vi "Climber Controller.vi"(8 "error in":errorcluster) -> ()   [LabVIEW 2019]
doc: "This VI executes continuously carrying out the current operation and responding to updates or new operations. It will often contain the timing or control code that is difficult to place directly in TeleOp. This VI generally opens all sensors and motors and isolates the rest of the robot code from knowing how the operations are carried out."
uses:
  <vilib>/Rock Robotics/WPI/Framework/Completion Status.ctl
  Climber Setpoints.ctl
  Climber Operations.ctl
  <vilib>/Rock Robotics/WPI/MotorControl/WPI_MotorControlDeviceRef.ctl
  <vilib>/Rock Robotics/WPI/MotorControl/WPI_MotorControlType.ctl
  <vilib>/Rock Robotics/SystemInterfaces/DIO/FPGA_DIOPWMChannel.ctl
  <vilib>/Rock Robotics/WPI/PWM/WPI_PWMDeadband.ctl
  <vilib>/Rock Robotics/SystemInterfaces/DIO/FPGA_DIOChannel.ctl
  <vilib>/Rock Robotics/WPI/ThirdParty/REV Robotics/SPARK MAX/Typedef/Spark MAX Limit Direction.ctl
panel:
  in  "Max Reverse Speed":dbl=-0.1
  out "Applied Output":dbl
  out "Sensor Velocity":dbl
  in  "Smart Position":dbl=40.0
  out "Sensor Position":dbl=-0.11904771625995636
  in  "Interactive Values":T1
  out "Current\nCmd":string="Started at  21:27:06.976\n: Extend Climb,  S 0.0, D 0.000000"
  in  "Buttons":cluster{"Execute Cmd":bool, "Abort Cmd":bool}
  out "Command Timing":cluster{"Start Time (ms)":u32, "Iterations":i32}={"Start Time (ms)"=7212987, "Iterations"=0}
  out "Status":T3
  # "Interactive Command: You may fill in the settings for a command\nand schedule it with the Execute button. You can observe and abort\nany command while fine tuning the code for the controller."
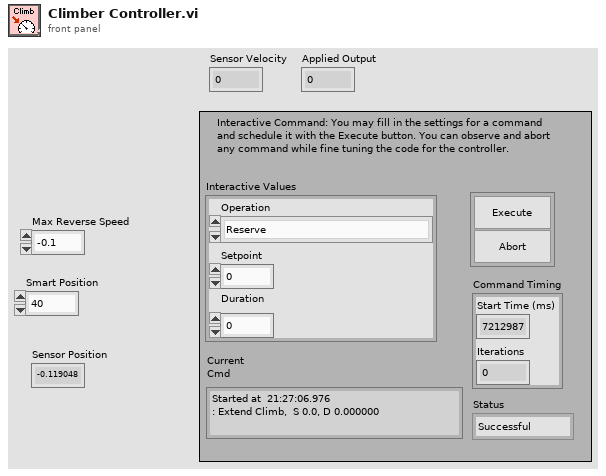
[diagram p1: front panel]
types:
  T1 = typedef "Climber Setpoints.ctl" = cluster{"Operation":T2, "Setpoint":dbl, "Duration":dbl}
  T2 = typedef "Climber Operations.ctl" = enum16{"Reserve", "Read Current", "Immediate", "Revert Climb", "Extend Climb"}
  T3 = typedef "Completion Status.ctl" = enum16{"Successful", "Aborted", "Incomplete"}
  T4 = typedef "Spark MAX Limit Direction.ctl" = enum16{"Forward Limit", "Reverse Limit"}
  T5 = typedef "WPI_MotorControlDeviceRef.ctl" = cluster{"DeviceStatus":errorcluster, "Type":T6, "PWM":cluster{"PWM Channel":T7, "DeadBand":T8}, "CAN":cluster{"Device Number":u8, "SetOutput VI Ref":variant, "GetOutput VI Ref":variant, "Enable VI Ref":variant, "Disable VI Ref":variant, "Data":variant}, "Invert":bool, "DIO PWM":cluster{"PWM \"Enable\" Channel":T7, "DIOChannel":T9, "PWM Rate":dbl}}
  T6 = typedef "WPI_MotorControlType.ctl" = enum16{"PWM", "CAN", "DIO PWM"}
  T7 = typedef "FPGA_DIOPWMChannel.ctl" = enum8{"PWM 0", "PWM 1", "PWM 2", "PWM 3", "PWM 4", "PWM 5", "PWM 6", "PWM 7", "PWM 8", "PWM 9", "PWM MXP 0", "PWM MXP 1", "PWM MXP 2", "PWM MXP 3", "PWM MXP 4", "PWM MXP 5", "PWM MXP 6", "PWM MXP 7", "PWM MXP 8", "PWM MXP 9", "Invalid"}
  T8 = typedef "WPI_PWMDeadband.ctl" = cluster{"Name":string, "maxPositivePwm":i32, "minPositivePwm":i32, "centerPwm":i32, "maxNegativePwm":i32, "minNegativePwm":i32, "angularRange":u16}
  T9 = typedef "FPGA_DIOChannel.ctl" = enum8{"DIO 0", "DIO 1", "DIO 2", "DIO 3", "DIO 4", "DIO 5", "DIO 6", "DIO 7", "DIO 8", "DIO 9", "DIO MXP 0", "DIO MXP 1", "DIO MXP 2", "DIO MXP 3", "DIO MXP 4", "DIO MXP 5", "DIO MXP 6", "DIO MXP 7", "DIO MXP 8", "DIO MXP 9", "DIO MXP 10", "DIO MXP 11", "DIO MXP 12", "DIO MXP 13", "DIO MXP 14", "DIO MXP 15", "SPI Port CS1", "SPI Port CS2", "SPI Port CS3", "SPI Port MISO", "SPI Port MOSI", "Invalid"}
  T10 = typedef "Command Status Info.ctl" = cluster{"Name":string, "Status":T3, "notifier out":T11}
  T11 = typedef "Completion Notifier.ctl" = refnum<notifier>
  T12 = cluster{"Current Command":T1, "Command Timing":cluster{"Start Time (ms)":u32, "Iterations":i32}, "Command Arguments":cluster{"Command Info":T10, "Description":string, "Default Command":T1, "queue out":refnum<queue>, "Subsystem Name":string}}
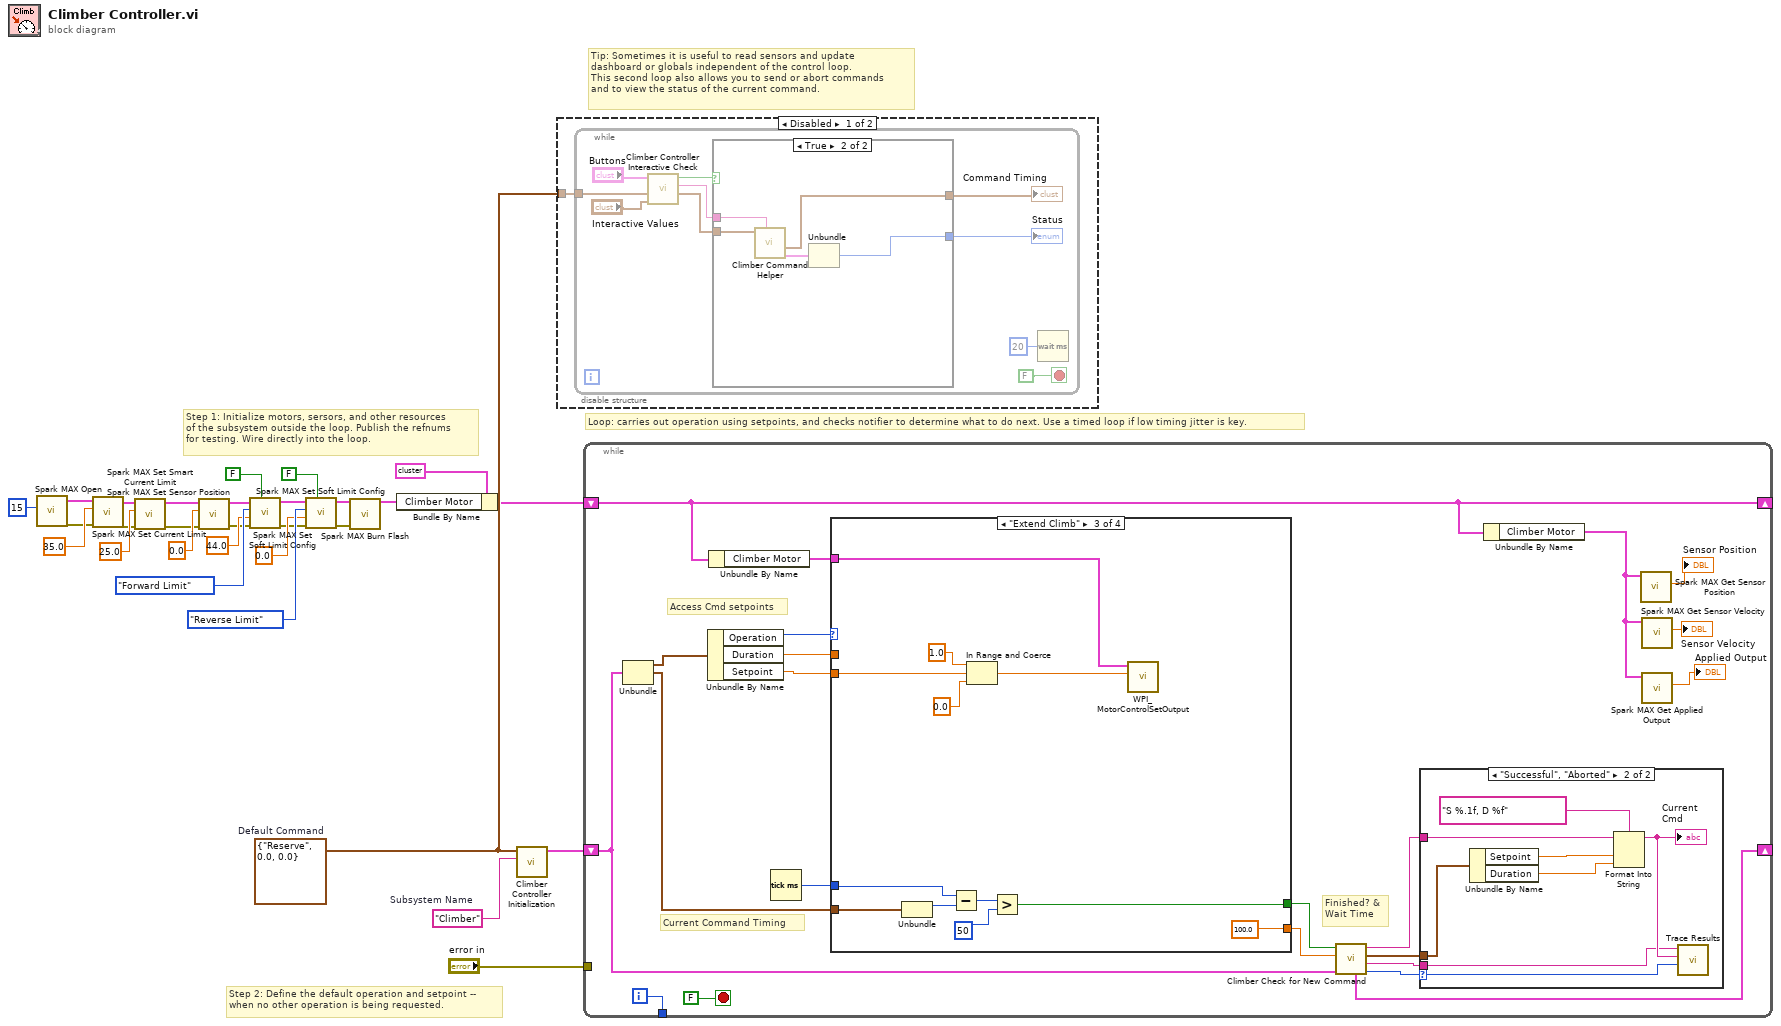
[diagram p0: block diagram]
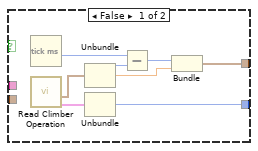
[diagram p2: hidden frame]
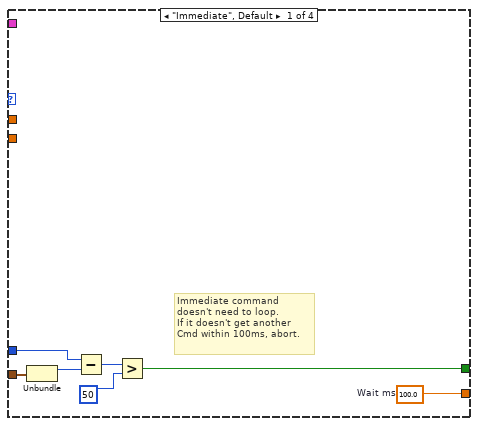
[diagram p5: hidden frame]
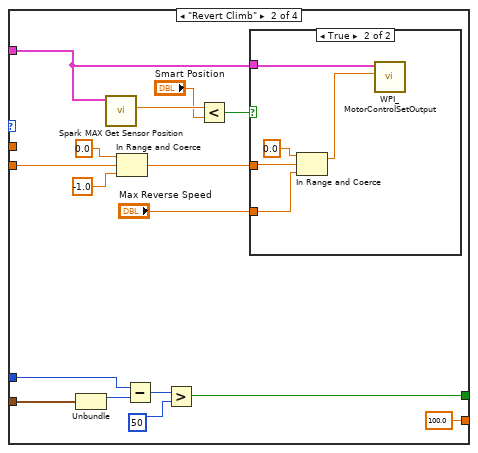
[diagram p6: hidden frame]
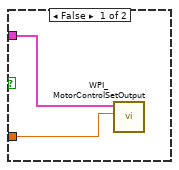
[diagram p7: hidden frame]
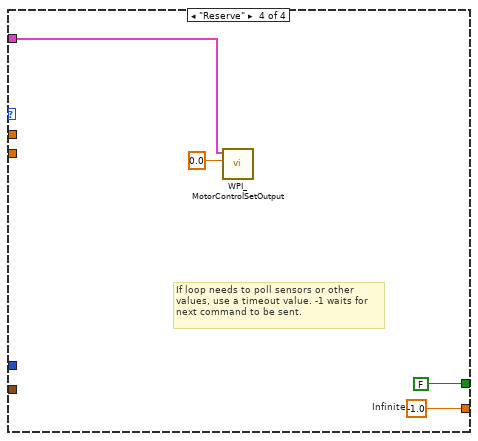
[diagram p8: hidden frame]
diagram:
  w26 = T1 {"Operation"=enum."Reserve", "Setpoint"=0.0, "Duration"=0.0}  # Default Command
  w27 = "Climber"  # Subsystem Name
  # "Tip: Sometimes it is useful to read sensors and update\ndashboard or globals independent of the control loop.\nThis second loop also allows you to send or abort commands\nand to view the status of the current command."
  # "Step 2: Define the default operation and setpoint --\nwhen no other operation is being requested."
  # "Step 1: Initialize motors, sersors, and other resources\nof the subsystem outside the loop. Publish the refnums\nfor testing. Wire directly into the loop."
  # "Loop: carries out operation using setpoints, and checks notifier to determine what to do next. Use a timed loop if low timing jitter is key."
  n1 = call <vilib>:"Spark MAX Open.vi"("Device Number"=u8 15) -> ("error out"=w3:errorcluster, "MotorControlDeviceRef"=w22:T5)  [unwired: 9 in]
  n2 = call <vilib>:"Spark MAX Set Current Limit.vi"("error in (no error)"=w3, "Current Limit A (100)"=sgl 35.0, "MotorControlDeviceRef in"=w22) -> ("error out"=w4:errorcluster, "MotorControlDeviceRef out"=w20:T5)  [unwired: 7 in]
  n3 = call <vilib>:"Spark MAX Set Smart Current Limit.vi"("error in (no error)"=w4, "Primay Current Limit (80A)"=25.0, "MotorControlDeviceRef in"=w20) -> ("error out"=w5:errorcluster, "MotorControlDeviceRef out"=w17:T5)  [unwired: 7 in]
  n4 = call <vilib>:"Spark MAX Set Sensor Position.vi"("error in"=w5, "Position"=0.0, "MotorControlDeviceRef"=w17) -> ("error out"=w6:errorcluster, "MotorControlDeviceRef"=w16:T5)  [unwired: 7 in]
  n5 = call <vilib>:"Spark MAX Set Soft Limit Config.vi"("Enabled? (T)"=FALSE, "error in (no error)"=w6, "Soft Limit (0)"=44.0, "Soft Limit Switch"=Spark_MAX_Limit_Direction."Forward Limit", "MotorControlDeviceRef in"=w16) -> ("error out"=w7:errorcluster, "MotorControlDeviceRef out"=w14:T5)  [unwired: 5 in]
  n6 = call <vilib>:"Spark MAX Set Soft Limit Config.vi"("Enabled? (T)"=FALSE, "error in (no error)"=w7, "Soft Limit (0)"=0.0, "Soft Limit Switch"=Spark_MAX_Limit_Direction."Reverse Limit", "MotorControlDeviceRef in"=w14) -> ("error out"=w10:errorcluster, "MotorControlDeviceRef out"=w9:T5)  [unwired: 5 in]
  n7 = call <vilib>:"Spark MAX Burn Flash.vi"("error in"=w10, "MotorControlDeviceRef"=w9) -> ("MotorControlDeviceRef"=w8:T5)  [unwired: 8 in, 1 out]
  n8 = Bundle By Name(cluster=cluster{"Climber Motor":T5} {"Climber Motor"={"DeviceStatus"={"status"=FALSE, "code"=0, "source"=""}, "Type"=enum."PWM", "PWM"={"PWM Channel"=enum."Invalid", "DeadBand"={"Name"="", "maxPositivePwm"=0, "minPositivePwm"=0, "centerPwm"=0, "maxNegativePwm"=0, "minNegativePwm"=0, "angularRange"=0}}, "CAN"={"Device Number"=0, "SetOutput VI Ref"=variant, "GetOutput VI Ref"=variant, "Enable VI Ref"=variant, "Disable VI Ref"=variant, "Data"=variant}, "Invert"=FALSE, "DIO PWM"={"PWM \"Enable\" Channel"=enum."Invalid", "DIOChannel"=enum."Invalid", "PWM Rate"=0.0}}} ("input cluster"), "Climber Motor"=w8) -> (w23:cluster{"Climber Motor":T5})
  n9 = call "Climber Controller Initialization.vi"("Subsystem Name"=w27, "Default Command"=w26) -> ("Current Command"=w28:T12)  [unwired: 9 in]
  n10 = disable-structure shown="Disabled" {
    disable-tunnel: w26 -> [w30 _]
    frame Disabled {
      n11 = while {
        tunnel: w30 -> [w37]
        stop <- FALSE stop-if-true
        n12 = call "Climber Controller Interactive Check.vi"("Interactive Command in"="Interactive Values", "Default Command"=w37, "Buttons"="Buttons") -> ("Interactive Command out"=w34:T1, "Trace String"=w35:string, "Schedule"=w36:bool)  [unwired: 6 in]
        n13 = case shown="True" w36 {
          tunnel: [w48 w53] -> w33
          tunnel: w34 -> [_ w51]
          tunnel: [w44 w49] -> w32
          tunnel: w35 -> [_ w52]
          frame False {
            n14 = Tick Count (ms)() -> (millisecond timer value=w43:u32)
            n15 = call "Read Climber Operation.vi"() -> ("Command Info"=w41:T10, "SubSystem Data"=w42:T1)  [unwired: 9 in, 1 out]
            n16 = Unbundle(w42) -> ("Operation"=w47:T2, "Setpoint"=w45:dbl)  [unwired: 1 out]
            n17 = Unbundle(w41) -> ("Status"=w48:T3)  [unwired: 2 out]
            n18 = Subtract(x=w43, y=w47) -> (x-y=w46:u32)
            n19 = Bundle(w46, "Setpoint"=w45) -> (w44:cluster{u32, "Setpoint":dbl})  [unwired: 1 in]
          }
          frame True {
            n20 = call "Climber Command Helper.vi"("Description"=w52, "SubSystem Data"=w51) -> ("Command Info Out"=w50:T10, "Command Timing"=w49:cluster{"Start Time (ms)":u32, "Iterations":i32})  [unwired: 7 in, 1 out]
            n21 = Unbundle(w50) -> ("Status"=w53:T3)  [unwired: 2 out]
          }
        }
        "Status" <- w33
        "Command Timing" <- w32
        n22 = Wait (ms)(milliseconds to wait=u32 20) -> ()  [unwired: 1 out]
      }
    }
    frame Enabled {
    }
  }
  n23 = while {
    shift-right: [w67] -> _
    shift-left: w28 -> [w60]
    tunnel: [w74] -> _
    tunnel: "error in" -> [_]
    shift-right: [w55] -> _
    shift-left: w23 -> [w55]
    i -> [w74]
    stop <- FALSE stop-if-true
    # "Current Command Timing"
    # "Access Cmd setpoints"
    # "Finished? &\nWait Time"
    n24 = Unbundle(w60) -> ("Current Command"=w73:T1, "Command Timing"=w69:cluster{"Start Time (ms)":u32, "Iterations":i32})  [unwired: 1 out]
    n25 = Unbundle By Name(w73) -> ("Operation"=w72:T2, "Duration"=w71:dbl, "Setpoint"=w68:dbl)
    n26 = Unbundle By Name(w55) -> ("Climber Motor"=w57:T5)
    n27 = Tick Count (ms)() -> (millisecond timer value=w70:u32)
    n28 = case shown="\"Extend Climb\"" w72 {
      tunnel: [w90 100.0 ("Infinite") 100.0 ("Infinite") w129] -> w65
      tunnel: [w84 w95 w117 FALSE ("ignore previous (F)")] -> w66
      tunnel: w69 -> [w86 w96 w119 _]
      tunnel: w71 -> [_ _ _ _]
      tunnel: w70 -> [w85 w97 w118 _]
      tunnel: w68 -> [_ w105 w123 _]
      tunnel: w57 -> [_ w104 w124 w127]
      frame "Immediate", Default {
        w90 = 100.0  # Wait ms
        # "Immediate command\ndoesn't need to loop.\nIf it doesn't get another\nCmd within 100ms, abort."
        n29 = Unbundle(w86) -> ("Start Time (ms)"=w89:u32)  [unwired: 1 out]
        n30 = Subtract(x=w85, y=w89) -> (x-y=w88:u32)
        n31 = Greater?(x=w88, y=u8 50 ("Left Motor")) -> (0:w84:bool)
      }
      frame "Revert Climb" {
        n32 = Unbundle(w96) -> ("Start Time (ms)"=w100:u32)  [unwired: 1 out]
        n33 = call <vilib>:"Spark MAX Get Sensor Position.vi"("MotorControlDevRef in"=w104) -> ("Sensor Position"=w102:dbl)  [unwired: 7 in, 3 out]
        n34 = In Range and Coerce(upper limit=0.0, x=w105, lower limit=-1.0) -> (coerced(x)=w93:dbl)  [unwired: 1 out]
        n35 = Subtract(x=w97, y=w100) -> (x-y=w99:u32)
        n36 = Greater?(x=w99, y=u8 50 ("Left Motor")) -> (0:w95:bool)
        n37 = Less?(x=w102, y="Smart Position") -> (x < y?=w103:bool)
        n38 = case shown="True" w103 {
          tunnel: w93 -> [w107 w112]
          tunnel: w104 -> [w108 w113]
          tunnel: "Max Reverse Speed" -> [_ w109]
          frame False {
            n39 = call <vilib>:"WPI_MotorControlSetOutput.vi"("Output"=w107, "MotorControlDevRef"=w108) -> ()  [unwired: 7 in, 3 out]
          }
          frame True {
            n40 = In Range and Coerce(upper limit=0.0, x=w112, lower limit=w109) -> (coerced(x)=w110:dbl)  [unwired: 1 out]
            n41 = call <vilib>:"WPI_MotorControlSetOutput.vi"("Output"=w110, "MotorControlDevRef"=w113) -> ()  [unwired: 7 in, 3 out]
          }
        }
      }
      frame "Extend Climb" {
        n42 = Unbundle(w119) -> ("Start Time (ms)"=w122:u32)  [unwired: 1 out]
        n43 = Subtract(x=w118, y=w122) -> (x-y=w121:u32)
        n44 = In Range and Coerce(upper limit=1.0, x=w123, lower limit=0.0) -> (coerced(x)=w116:dbl)  [unwired: 1 out]
        n45 = Greater?(x=w121, y=u8 50 ("Left Motor")) -> (0:w117:bool)
        n46 = call <vilib>:"WPI_MotorControlSetOutput.vi"("Output"=w116, "MotorControlDevRef"=w124) -> ()  [unwired: 7 in, 3 out]
      }
      frame "Reserve" {
        w129 = -1.0  # Infinite
        # "If loop needs to poll sensors or other\nvalues, use a timeout value. -1 waits for\nnext command to be sent."
        n47 = call <vilib>:"WPI_MotorControlSetOutput.vi"("Output"=0.0, "MotorControlDevRef"=w127) -> ()  [unwired: 7 in, 3 out]
      }
    }
    n48 = call "Climber Check for New Command.vi"("Current Command"=w60, "Wait time (ms)"=w65, "Finished?"=w66) -> ("Completion"=w61:T3, "Subsystem Name"=w62:string, "Current Command"=w63:T1, "Initial Trace String"=w64:string, "NextCommand"=w67:T12)  [unwired: 4 in]
    n49 = case shown="\"Successful\", \"Aborted\"" w61 {
      selector: w61 -> [_ w83]
      tunnel: w64 -> [_ w79]
      tunnel: w63 -> [_ w80]
      tunnel: w62 -> [_ w76]
      frame "Incomplete", Default {
        # "Continuing current command"
      }
      frame "Successful", "Aborted" {
        # "Report and setup for next command"
        n50 = Unbundle By Name(w80) -> ("Setpoint"=w82:dbl, "Duration"=w77:dbl)
        n51 = Format Into String(format string="S %.1f, D %f", initial string=w79, w82, w77) -> (resulting string=w78:string)  [unwired: 1 in, 1 out]
        "Current\nCmd" <- w78
        n52 = call <vilib>:"Trace Results.vi"("Status of previous command"=w83, "Description"=w78, "Subsystem"=w76) -> ()  [unwired: 9 in]
      }
    }
    n53 = Unbundle By Name(w55) -> ("Climber Motor"=w54:T5)
    n54 = call <vilib>:"Spark MAX Get Sensor Position.vi"("MotorControlDevRef in"=w54) -> ("Sensor Position"=→"Sensor Position":dbl)  [unwired: 7 in, 3 out]
    n55 = call <vilib>:"Spark MAX Get Sensor Velocity.vi"("MotorControlDevRef in"=w54) -> ("Sensor Velocity"=→"Sensor Velocity":dbl)  [unwired: 7 in, 3 out]
    n56 = call <vilib>:"Spark MAX Get Applied Output.vi"("MotorControlDevRef in"=w54) -> ("Applied Output"=→"Applied Output":dbl)  [unwired: 7 in, 3 out]
  }
